vi "update_version.vi"(8 "error in (no error)":errorcluster, 9 "commit_hash":string, 10 "version":string, 11 "version_vi":path) -> (0 "error out":errorcluster)   [LabVIEW 2015, in "lv-builder.lvlib"]
uses:
  lv-builder.lvlib
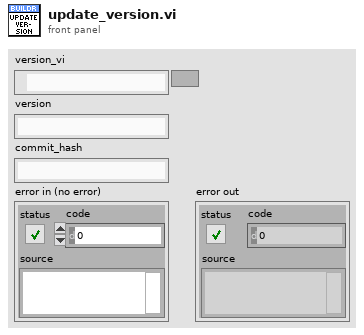
[diagram p1: front panel]
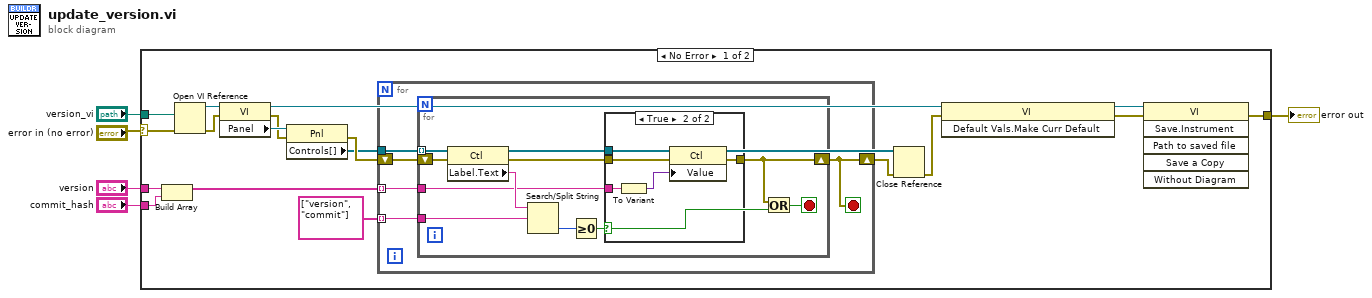
[diagram p0: block diagram]
diagram:
  n1 = case shown="No Error" "error in (no error)" {
    selector: "error in (no error)" -> [w19 w46]
    tunnel: [w15 w46] -> w5
    tunnel: "version_vi" -> [w20 _]
    tunnel: "version" -> [w12 _]
    tunnel: "commit_hash" -> [w11 _]
    frame No Error {
      n2 = Build Array(w12, w11) -> (w10:string[])
      n3 = Open VI Reference(vi path=w20, error in (no error)=w19) -> (vi reference=w14:refnum<vi>, error out=w13:errorcluster)  [unwired: 4 in]
      n4 = property class="VI"(reference=w14, error in=w13) -> (reference out=w18:refnum<vi>, error out=w22:errorcluster, "Panel"=w23:refnum<vi>)
      n5 = property class="Pnl"(reference=w23, error in=w22) -> (error out=w21:errorcluster, "Controls[]"=w8:refnum<vi>[])  [unwired: 1 out]
      n6 = for {
        tunnel: w8 -> [w28]
        tunnel: w10 -> [w26] mode=indexing
        tunnel: string[] ["version", "commit"] -> [w25] mode=indexing
        shift-right: [w24] -> w7
        shift-left: w21 -> [w27]
        stop <- w24 stop-if-true
        n7 = for {
          tunnel: w28 -> [w39] mode=indexing
          shift-right: [w33] -> w24
          shift-left: w27 -> [w34]
          tunnel: w26 -> [w31]
          tunnel: w25 -> [w30]
          stop <- w29 stop-if-true
          n8 = property class="Ctl"(reference=w39, error in=w34) -> (reference out=w36:refnum<vi>, error out=w35:errorcluster, "Label.Text"=w38:string)
          n9 = Search/Split String(string=w38, search string/char (-)=w30) -> (offset of match=w37:i32)  [unwired: 1 in, 2 out]
          n10 = Greater Or Equal To 0?(x=w37) -> (x >= 0?=w32:bool)
          n11 = case shown="True" w32 {
            tunnel: w36 -> [_ w45]
            tunnel: w35 -> [w40 w44]
            tunnel: [w40 w43] -> w33
            tunnel: w31 -> [_ w41]
            frame False {
            }
            frame True {
              n12 = To Variant(anything=w41) -> (Variant=w42:variant)
              n13 = property class="Ctl"(reference=w45, error in=w44, "Value"=w42) -> (error out=w43:errorcluster)  [unwired: 1 out]
            }
          }
          n14 = Or(x=w33, y=w32) -> (x .or. y?=w29:bool)
        }
      }
      n15 = Close Reference(reference=w8, error in (no error)=w7) -> (error out=w6:errorcluster)
      n16 = invoke class="VI" method="Default Vals.Make Curr Default"(reference=w18, error in=w6) -> (reference out=w16:refnum<vi>, error out=w17:errorcluster)  [unwired: 1 in, 1 out]
      n17 = invoke class="VI" method="Save.Instrument"(reference=w16, error in=w17) -> (error out=w15:errorcluster)  [unwired: 4 in, 5 out]
    }
    frame Error {
    }
  }
  "error out" <- w5
